vi "HTML.vi"() -> ()   [LabVIEW 2020]
uses:
  C:/Data/WebBrowser/WebBrowser/packages/Microsoft.Web.WebView2.1.0.864.35/Microsoft.Web.WebView2.1.0.864.35/lib/net45/Microsoft.Web.WebView2.WinForms.dll
  Data/WebBrowser/WebBrowser/packages/Microsoft.Web.WebView2.1.0.864.35/Microsoft.Web.WebView2.1.0.864.35/lib/net45/Microsoft.Web.WebView2.WinForms.dll
panel:
  in  "WebView2":refnum<k24>(container)
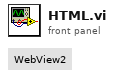
[diagram p1: front panel]
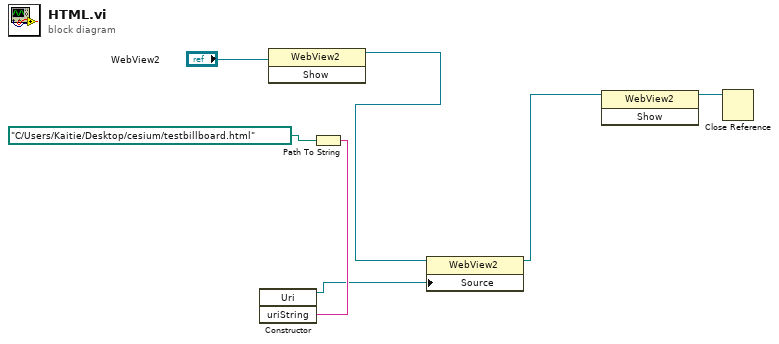
[diagram p0: block diagram]
diagram:
  n1 = invoke class="WebView2" method="Show"(reference="WebView2") -> (reference out=w1:refnum<k24>)  [unwired: 2 in, 2 out]
  n2 = Path To String(path=path "C:/Users/Kaitie/Desktop/cesium/testbillboard.html") -> (string=w6:string)
  n3 = constructor class="Uri"("uriString"=w6) -> (reference out=w5:refnum<k24>)  [unwired: 3 in, 3 out]
  n4 = property class="WebView2"(reference=w1, "Source"=w5) -> (reference out=w4:refnum<k24>)  [unwired: 1 in, 1 out]
  n5 = invoke class="WebView2" method="Show"(reference=w4) -> (reference out=w3:refnum<k24>)  [unwired: 2 in, 2 out]
  n6 = Close Reference(reference=w3) -> ()  [unwired: 1 in, 1 out]
